vi "Enable Next.vi"(9 "Spec Page Interface":T1, 10 "Supported Data Types":refnum<vi>, 11 "ListBox in":refnum<vi>) -> ()   [LabVIEW 2013, in "DCAFConfigurablePluginDecideFeatures.lvclass"]
uses:
  DCAFConfigurablePluginDecideFeatures.lvclass
  <resource>/dialog/NewProjectWizard/Spec Page Interface.ctl
  Button Names.ctl
panel:
  out "error out":errorcluster
  in  "error in (no error)":errorcluster
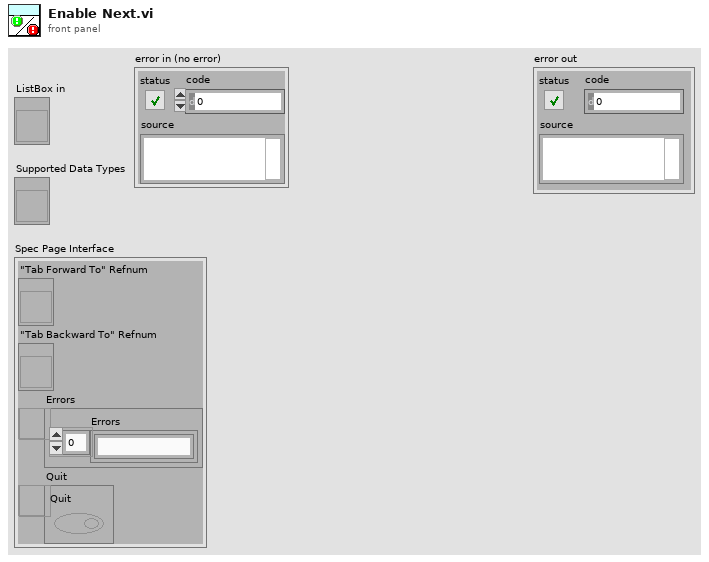
[diagram p1: front panel]
types:
  T1 = typedef "Spec Page Interface.ctl" = cluster{"\"Tab Forward To\" Refnum":refnum<vi>, "\"Tab Backward To\" Refnum":refnum<vi>, "Errors":refnum<user-event>, "Quit":refnum<user-event>}
  T2 = enum8{"Enabled", "Disabled", "Disabled and Grayed Out"}
  T3 = typedef "Button Names.ctl" = enum16{"Back", "Next", "Help", "Cancel"}
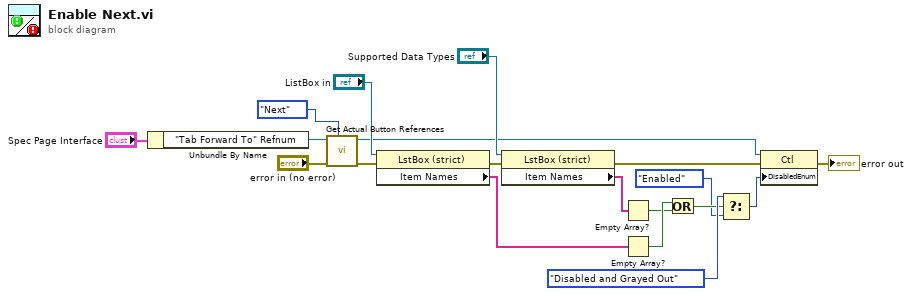
[diagram p0: block diagram]
diagram:
  n1 = Unbundle By Name("Spec Page Interface") -> ("\"Tab Forward To\" Refnum"=w12:refnum<vi>)
  n2 = call "Get Actual Button References.vi"("Enum"=Button_Names."Next", "error in (no error)"="error in (no error)", "\"Tab Forward To\" Refnum"=w12) -> ("error out"=w2:errorcluster, "Refnum out"=w10:refnum<vi>)  [unwired: 7 in]
  n3 = property on="Property Node" class="LstBox (strict)"(reference="ListBox in", error in=w2) -> (error out=w4:errorcluster, "Item Names"=w16:string[])  [unwired: 1 out]
  n4 = property class="LstBox (strict)"(reference="Supported Data Types", error in=w4) -> (error out=w5:errorcluster, "Item Names"=w17:string[])  [unwired: 1 out]
  n5 = Empty Array?(array=w17) -> (empty?=w18:bool)
  n6 = Empty Array?(array=w16) -> (empty?=w19:bool)
  n7 = Or(x=w19, y=w18) -> (x .or. y?=w8:bool)
  n8 = Select(t=T2."Disabled and Grayed Out" ("Disabled"), s=w8, f=T2."Enabled") -> (s? t:f=w1:T2)
  n9 = property class="Ctl"(reference=w10, error in=w5, "DisabledEnum"=w1) -> (error out=→"error out":errorcluster)  [unwired: 1 out]
